vi "Decrement ShotCounter.vi"(8 "error in (no error)":errorcluster, 11 "HIJ Vision Camera App w Timer in":refnum<class "HIJ Vision Camera App w Timer.lvclass">) -> (0 "error out":errorcluster, 3 "HIJ Vision Camera App w Timer out":refnum<class "HIJ Vision Camera App w Timer.lvclass">)   [LabVIEW 2014, in "HIJ Vision Camera App w Timer.lvlib" / "HIJ Vision Camera App w Timer.lvclass"]
uses:
  HIJ Vision Camera App w Timer.lvclass
  HIJ Vision Camera App w Timer.lvclass/HIJ Vision Camera App w Timer.ctl
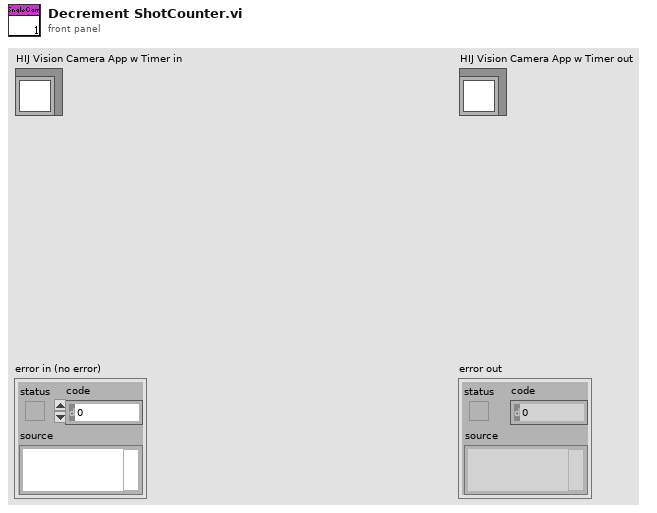
[diagram p1: front panel]
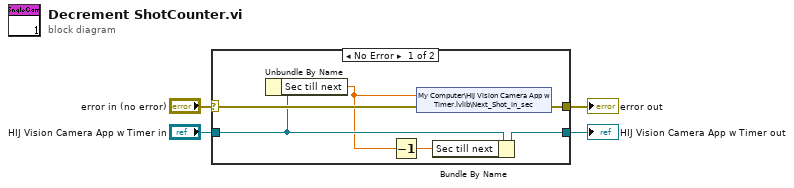
[diagram p0: block diagram]
diagram:
  n1 = case shown="No Error" "error in (no error)" {
    selector: "error in (no error)" -> [w10 w12]
    tunnel: [w9 w12] -> w3
    tunnel: [w7 w11] -> w1
    tunnel: "HIJ Vision Camera App w Timer in" -> [w8 w11]
    frame No Error {
      n2 = Unbundle By Name(w8) -> ("Sec till next"=w6:dbl)
      n3 = Decrement(x=w6) -> (x-1=w5:dbl)
      n4 = shared-variable "My Computer\\HIJ Vision Camera App w Timer.lvlib\\Next_Shot_in_sec"(w6, error in=w10) -> (error out=w9:errorcluster)
      n5 = Bundle By Name(cluster=w8, "Sec till next"=w5) -> (w7:refnum<class "HIJ Vision Camera App w Timer.lvclass">)
    }
    frame Error {
    }
  }
  "error out" <- w3
  "HIJ Vision Camera App w Timer out" <- w1
